vi "VarBRS.vi"(1 "A":dbl, 2 "C":dbl, 3 "A=0":bool, 4 "C=0":bool) -> (0 "BRS":dbl)   [LabVIEW 2012]
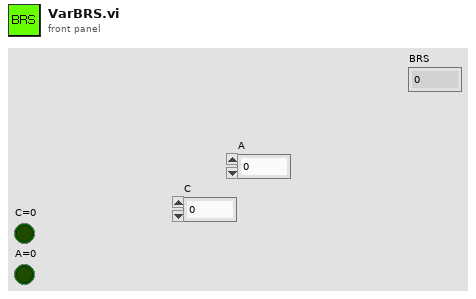
[diagram p1: front panel]
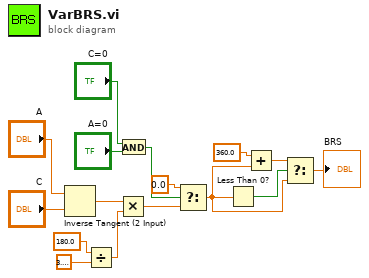
[diagram p0: block diagram]
diagram:
  n1 = Inverse Tangent (2 Input)(1:"C", 2:"A") -> (0:w9:dbl)
  n2 = Divide(x=180.0, y=3.141592653589793) -> (x/y=w10:dbl)
  n3 = Multiply(x=w9, y=w10) -> (x*y=w8:dbl)
  n4 = And(x="C=0", y="A=0") -> (x .and. y?=w14:bool)
  n5 = Select(t=0.0, s=w14, f=w8) -> (s? t:f=w2:dbl)
  n6 = Less Than 0?(x=w2) -> (x < 0?=w5:bool)
  n7 = Add(x=360.0, y=w2) -> (x+y=w4:dbl)
  n8 = Select(t=w4, s=w5, f=w2) -> (s? t:f=→"BRS":dbl)
